vi "Check_Ini_Log_File.vi"(0 "Application path":path, 1 "State":T1, 3 "error in (no error)":errorcluster) -> (5 "Application path":path, 7 "error out":errorcluster)   [LabVIEW 2023]
doc: "This VI searches for the datalog file if it doens't exists (FALSE case)\nit creates the file else it appends the info. to the already existing file"
uses:
  Controls/State.ctl
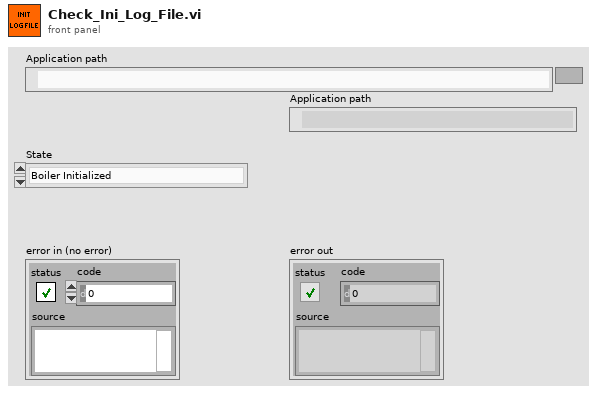
[diagram p1: front panel]
types:
  T1 = typedef "State.ctl" = enum16{"Boiler Initialized", "Boiler Ready", "Start Pre-Purge", "Pre-Purge Complete", "Pilot On", "Pilot Proved", "Force Draft Fan ON", "Shutdown and Purge", "Wait for Something"}
  T2 = enum16{"open", "replace", "create", "open or create", "replace or create", "replace or create with confirmation"}
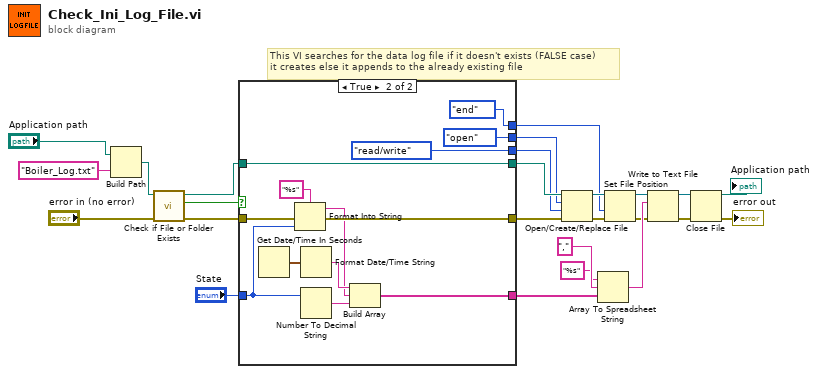
[diagram p0: block diagram]
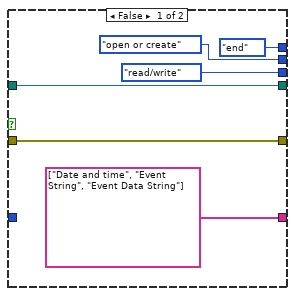
[diagram p2: hidden frame]
diagram:
  # "This VI searches for the data log file if it doesn't exists (FALSE case)\nit creates else it appends to the already existing file"
  n1 = Build Path(base path="Application path", name or relative path="Boiler_Log.txt") -> (appended path=w22:path)
  n2 = call <vilib>:"Check if File or Folder Exists.vi"("error in (no error)"="error in (no error)", "path"=w22) -> ("error out"=w24:errorcluster, "file or folder exists?"=w23:bool, "dup path"=w25:path)  [unwired: 7 in]
  n3 = case shown="True" w23 {
    tunnel: w24 -> [w31 w40]
    tunnel: w25 -> [w30 w44]
    tunnel: [w31 w39] -> w13
    tunnel: [w30 w44] -> w7
    tunnel: [T2."open or create" ("operation (0:open)") T2."open" ("operation (0:open)")] -> w6
    tunnel: [enum16{"read/write", "read-only", "write-only"}."read/write" ("access (0:read/write)") enum16{"read/write", "read-only", "write-only"}."read/write" ("access (0:read/write)")] -> w5
    tunnel: [string[] ["Date and time", "Event String", "Event Data String"] w35] -> w11
    tunnel: "State" -> [_ w33]
    tunnel: [enum16{"start", "end", "current"}."end" ("from (0:start)") enum16{"start", "end", "current"}."end" ("from (0:start)")] -> w4
    frame False {
    }
    frame True {
      n4 = Get Date/Time In Seconds() -> (seconds since 1Jan1904=w41:timestamp)
      n5 = Format Into String(format string="%s", error in=w40, w33) -> (resulting string=w36:string, error out=w39:errorcluster)  [unwired: 1 in]
      n6 = Format Date/Time String(seconds (now)=w41) -> (date/time string=w37:string)  [unwired: 2 in]
      n7 = Number To Decimal String(number=w33) -> (decimal integer string=w32:string)  [unwired: 1 in]
      n8 = Build Array(w37, w36, w32) -> (w35:string[])
    }
  }
  n9 = Open/Create/Replace File(file path (use dialog)=w7, error in=w13, operation (0:open)=w6, access (0:read/write)=w5) -> (refnum out=w16:refnum<file>, error out=w8:errorcluster)  [unwired: 2 in, 1 out]
  n10 = Array To Spreadsheet String(delimiter (Tab)=",", array=w11, 3:"%s" ("format string")) -> (spreadsheet string=w15:string)
  n11 = Set File Position(refnum=w16, from (0:start)=w4, error in=w8) -> (refnum out=w17:refnum<file>, error out=w3:errorcluster)  [unwired: 1 in]
  n12 = Write to Text File(file (use dialog)=w17, text=w15, error in=w3) -> (refnum out=w14:refnum<file>, error out=w2:errorcluster)  [unwired: 1 in, 1 out]
  n13 = Close File(refnum=w14, error in=w2) -> (path=→"Application path":path, error out=→"error out":errorcluster)
